vi "sub_conv_enc_v2.vi"(8 "code type":T1(ring)=enum."r=1/2 (13,17)", 11 "bitstream":i32[](array[numeric])) -> (3 "coded bits":i16[](array[numeric]))   [LabVIEW 2014]
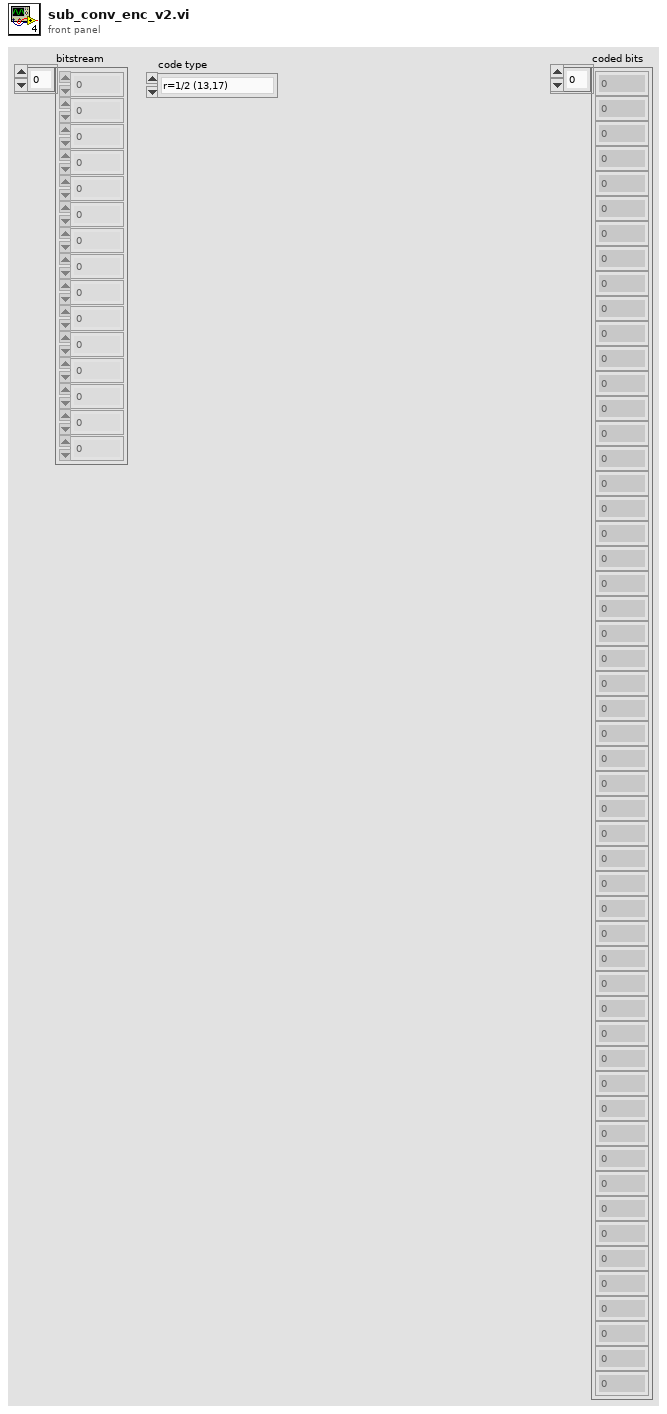
[diagram p1: front panel]
types:
  T1 = enum16{"r=1/2 (5,7)", "r=1/2 (13,17)", "r=1/4 (25,27,33,37)"}
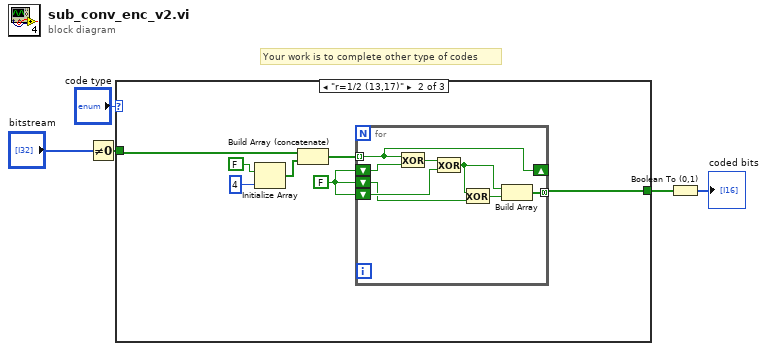
[diagram p0: block diagram]
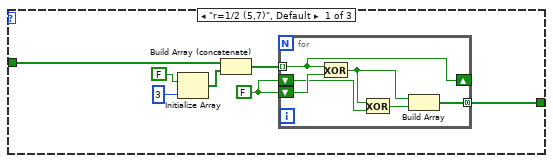
[diagram p2: hidden frame]
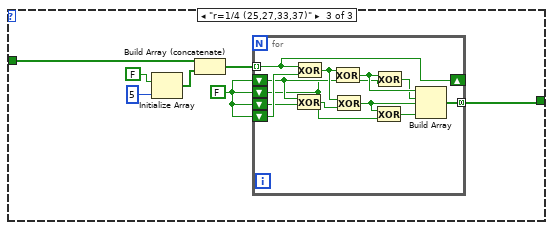
[diagram p3: hidden frame]
diagram:
  # "Your work is to complete other type of codes"
  n1 = Not Equal To 0?(x="bitstream") -> (x != 0?=w3:bool[])
  n2 = case shown="\"r=1/2 (13,17)\"" "code type" {
    tunnel: w3 -> [w8 w21 w36]
    tunnel: [w11 w20 w35] -> w2
    frame "r=1/2 (5,7)", Default {
      w12 = FALSE
      n3 = Initialize Array(FALSE, 3 ("dimension size")) -> (w7:bool[])
      n4 = Build Array (concatenate)(w8, w7) -> (w6:bool[])
      n5 = for {
        tunnel: w6 -> [w13] mode=indexing
        shift-right: [w13] -> _
        shift-left: w12 -> [w15]
        shift-left: w12 -> [w17]
        tunnel: [w18] -> w11 mode=concatenating
        n6 = Exclusive Or(1:w17, 2:w13) -> (0:w16:bool)
        n7 = Exclusive Or(1:w15, 2:w16) -> (0:w14:bool)
        n8 = Build Array(w16, w14) -> (w18:bool[])
      }
    }
    frame "r=1/2 (13,17)" {
      w19 = FALSE
      n9 = Initialize Array(FALSE, 4 ("dimension size")) -> (w23:bool[])
      n10 = Build Array (concatenate)(w21, w23) -> (w22:bool[])
      n11 = for {
        tunnel: w22 -> [w32] mode=indexing
        shift-right: [w32] -> _
        shift-left: w19 -> [w31]
        shift-left: w19 -> [w29]
        tunnel: [w33] -> w20 mode=concatenating
        shift-left: w19 -> [w27]
        n12 = Exclusive Or(1:w31, 2:w32) -> (0:w30:bool)
        n13 = Exclusive Or(1:w29, 2:w30) -> (0:w28:bool)
        n14 = Exclusive Or(1:w27, 2:w28) -> (0:w26:bool)
        n15 = Build Array(w28, w26) -> (w33:bool[])
      }
    }
    frame "r=1/4 (25,27,33,37)" {
      w34 = FALSE
      n16 = Initialize Array(FALSE, 5 ("dimension size")) -> (w38:bool[])
      n17 = Build Array (concatenate)(w36, w38) -> (w37:bool[])
      n18 = for {
        tunnel: w37 -> [w49] mode=indexing
        shift-right: [w49] -> _
        shift-left: w34 -> [w44]
        shift-left: w34 -> [w47]
        tunnel: [w52] -> w35 mode=concatenating
        shift-left: w34 -> [w41]
        shift-left: w34 -> [w48]
        n19 = Exclusive Or(1:w47, 2:w44) -> (0:w46:bool)
        n20 = Exclusive Or(1:w48, 2:w49) -> (0:w45:bool)
        n21 = Exclusive Or(1:w41, 2:w45) -> (0:w51:bool)
        n22 = Exclusive Or(1:w46, 2:w45) -> (0:w42:bool)
        n23 = Exclusive Or(1:w41, 2:w42) -> (0:w43:bool)
        n24 = Exclusive Or(1:w44, 2:w51) -> (0:w50:bool)
        n25 = Build Array(w51, w50, w42, w43) -> (w52:bool[])
      }
    }
  }
  n26 = Boolean To (0,1)(Boolean=w2) -> (0, 1=→"coded bits":i16[])
